vi "DAQ Parameters.vi"(7 "action":T1, 8 "error in":errorcluster, 10 "Sample Params Names IN":string[](array[string]), 11 "Run Params Names IN":string[](array[string])) -> (0 "error out":errorcluster, 2 "Sample Params Names OUT":string[](array[string]), 3 "Run Params Names OUT":string[](array[string]))   [LabVIEW 2011]
uses:
  DAQ Parameters.ctl
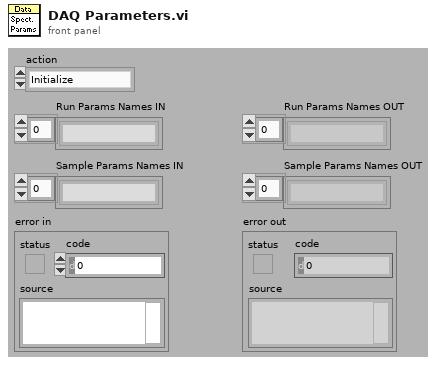
[diagram p1: front panel]
types:
  T1 = typedef "DAQ Parameters.ctl" = enum16{"Initialize", "Set Run Param Names", "Get Run Param Names", "Set Sample Param Names", "Get Sample Param Names"}
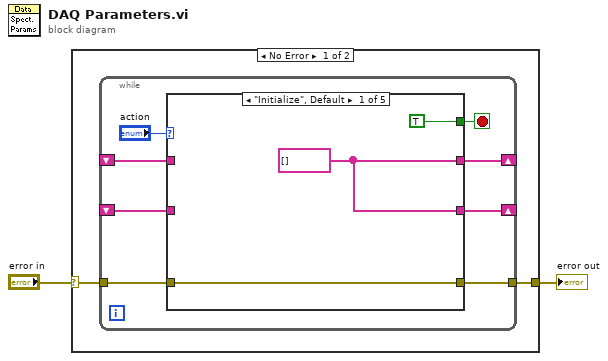
[diagram p0: block diagram]
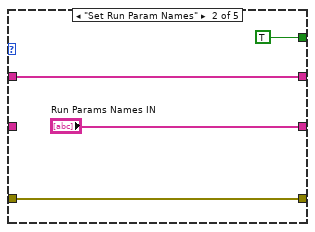
[diagram p2: hidden frame]
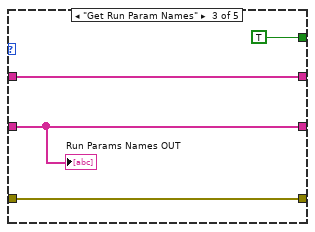
[diagram p3: hidden frame]
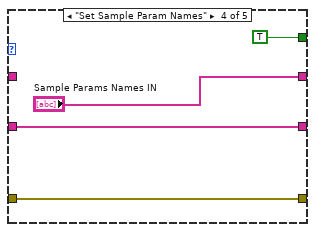
[diagram p4: hidden frame]
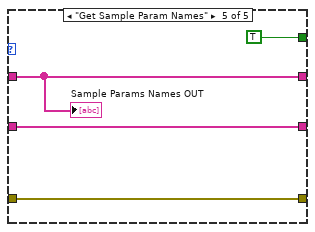
[diagram p5: hidden frame]
diagram:
  n1 = case shown="No Error" "error in" {
    selector: "error in" -> [w3 w32]
    tunnel: [w4 w32] -> w1
    frame No Error {
      n2 = while {
        shift-right: [w11] -> _
        shift-left: _ -> [w10]
        tunnel: [w9] -> w4
        tunnel: w3 -> [w8]
        shift-right: [w6] -> _
        shift-left: _ -> [w5]
        stop <- w7 stop-if-true
        n3 = case shown="\"Initialize\", Default" "action" {
          tunnel: [w13 w19 w23 "Sample Params Names IN" w29] -> w11
          tunnel: w10 -> [_ w19 w23 _ w29]
          tunnel: [w15 w17 w21 w26 w31] -> w9
          tunnel: w8 -> [w15 w17 w21 w26 w31]
          tunnel: [TRUE TRUE TRUE TRUE TRUE] -> w7
          tunnel: [w13 "Run Params Names IN" w22 w24 w28] -> w6
          tunnel: w5 -> [_ _ w22 w24 w28]
          frame "Initialize", Default {
            w13 = string[] [] ("Spectrum Params IN")
          }
          frame "Set Run Param Names" {
          }
          frame "Get Run Param Names" {
            "Run Params Names OUT" <- w22
          }
          frame "Set Sample Param Names" {
          }
          frame "Get Sample Param Names" {
            "Sample Params Names OUT" <- w29
          }
        }
      }
    }
    frame Error {
    }
  }
  "error out" <- w1
